vi "meas.vi"() -> ()   [LabVIEW 2010]
doc: "Use this template to create an application that executes until you click the Stop button. Unlike the Single Loop Application VI that uses polling, this VI uses the Event structure."
uses:
  <vilib>/Utility/config.llb/Read Key (String).vi
  <vilib>/Utility/config.llb/Read Key (Path).vi
  <vilib>/Utility/config.llb/Read Key (I32).vi
  <vilib>/Utility/config.llb/Read Key (Boolean).vi
  <vilib>/Utility/config.llb/Write Key (Boolean).vi
  <vilib>/Utility/config.llb/Write Key (I32).vi
  <vilib>/Utility/config.llb/Write Key (String).vi
  <vilib>/Utility/config.llb/Write Key (Path).vi
  <vilib>/Utility/config.llb/NI_LVConfig.lvlib
panel:
  in  "Export":bool
  in  "Trend":bool
  out "Array 2":u32[](array[colorbox])=[16711680, 16774656, 2783999, 65280]
  in  "MeasData":T1
  in  "Array":string[](array[string])
  in  "Tab Control":enum32{"Measurements", "View"}(tab)
  in  "Table":string[][](table)
  out "Q(R)":cluster{"Ph":i32[], dbl[]}[](graph)
  out "APD":cluster{"Ph":i32[], dbl[]}[](graph)
  out "Bar graph":cluster{"y_hist":i32[], "x_hist":i32[]}[](graph)
  out "Trend":cluster{i32[], i32[]}[](graph)
  out "Q(R)":cluster{"Ph":i32[], dbl[]}[](graph)
  out "Amplitude/Phaze":cluster{"Ph":i32[], dbl[]}[](graph)
  out "Histogram":cluster{"y_hist":i32[], "x_hist":i32[]}[](graph)
  out "ct":i32
  in  "Time delay":i32
  in  "NewFile":bool
  in  "Mesage":string(combo)
  out "Number of samples":i32
  out "ConTest":bool
  in  "VISA resource name":refnum<visa-resource-name>="ASRL1::INSTR"
  out "Connection test time":string caption="Connection test"
  in  "Stop":bool
  in  "OpenFile":bool
  in  "New":bool
  out "Object name":string
  out "File Path":path
  out "Slide":dbl(slide) scale=0.0..100.0
  in  "Auto":bool
  out "QR50":dbl[](array[numeric])
  # "Measuring"
  # "Qr50, pC"
  # "Ch 1"
  # "Ch 2"
  # "Ch 3"
  # "Ch 4"
  # "Auto"
  # "F i l e"
  # "Port name"
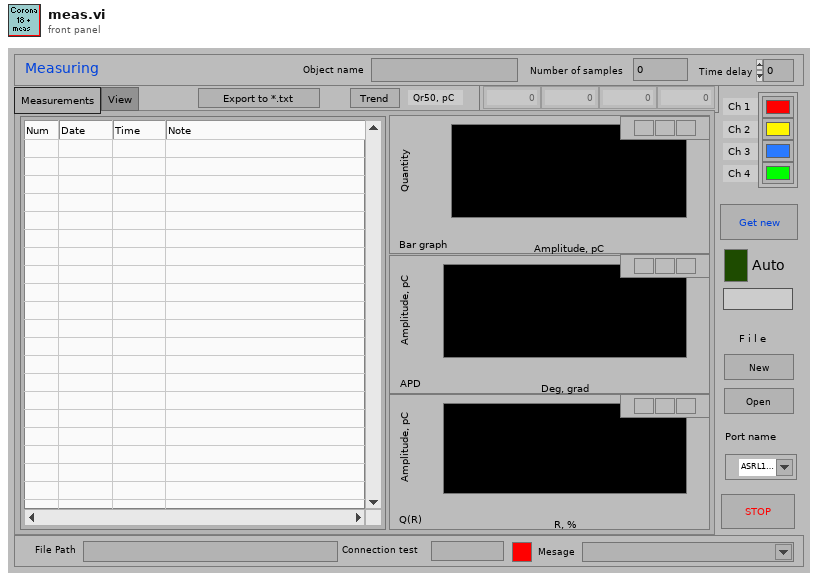
[diagram p1: front panel]
types:
  T1 = cluster{"Charge":i32, "U_Charge":i32[], "Shift":i32, "WinW":i32, "Qr":i32[][], "Ph":i32[][], "y_hist":i32[][], "x_hist":i32[][]}
  T2 = typedef "NI_LVConfig.lvlib/Config Data RefNum.ctl" = refnum<k1>
  T3 = cluster{"Array":string[], "MeasData":cluster{"Charge":i32, "U_Charge":i32[], "Shift":i32, "WinW":i32, "Qr":i32[][], "Ph":i32[][], "y_hist":i32[][], "x_hist":i32[][]}}[]
  T4 = typedef "LVRowAndColumnTypeDef.ctl" = cluster{"Row":i32, "Column":i32}
  T5 = cluster{"Array":string[], "MeasData":cluster{"Charge":i32, "U_Charge":i32[], "Shift":i32, "WinW":i32, "Qr":i32[][], "Ph":i32[][], "y_hist":i32[][], "x_hist":i32[][]}}
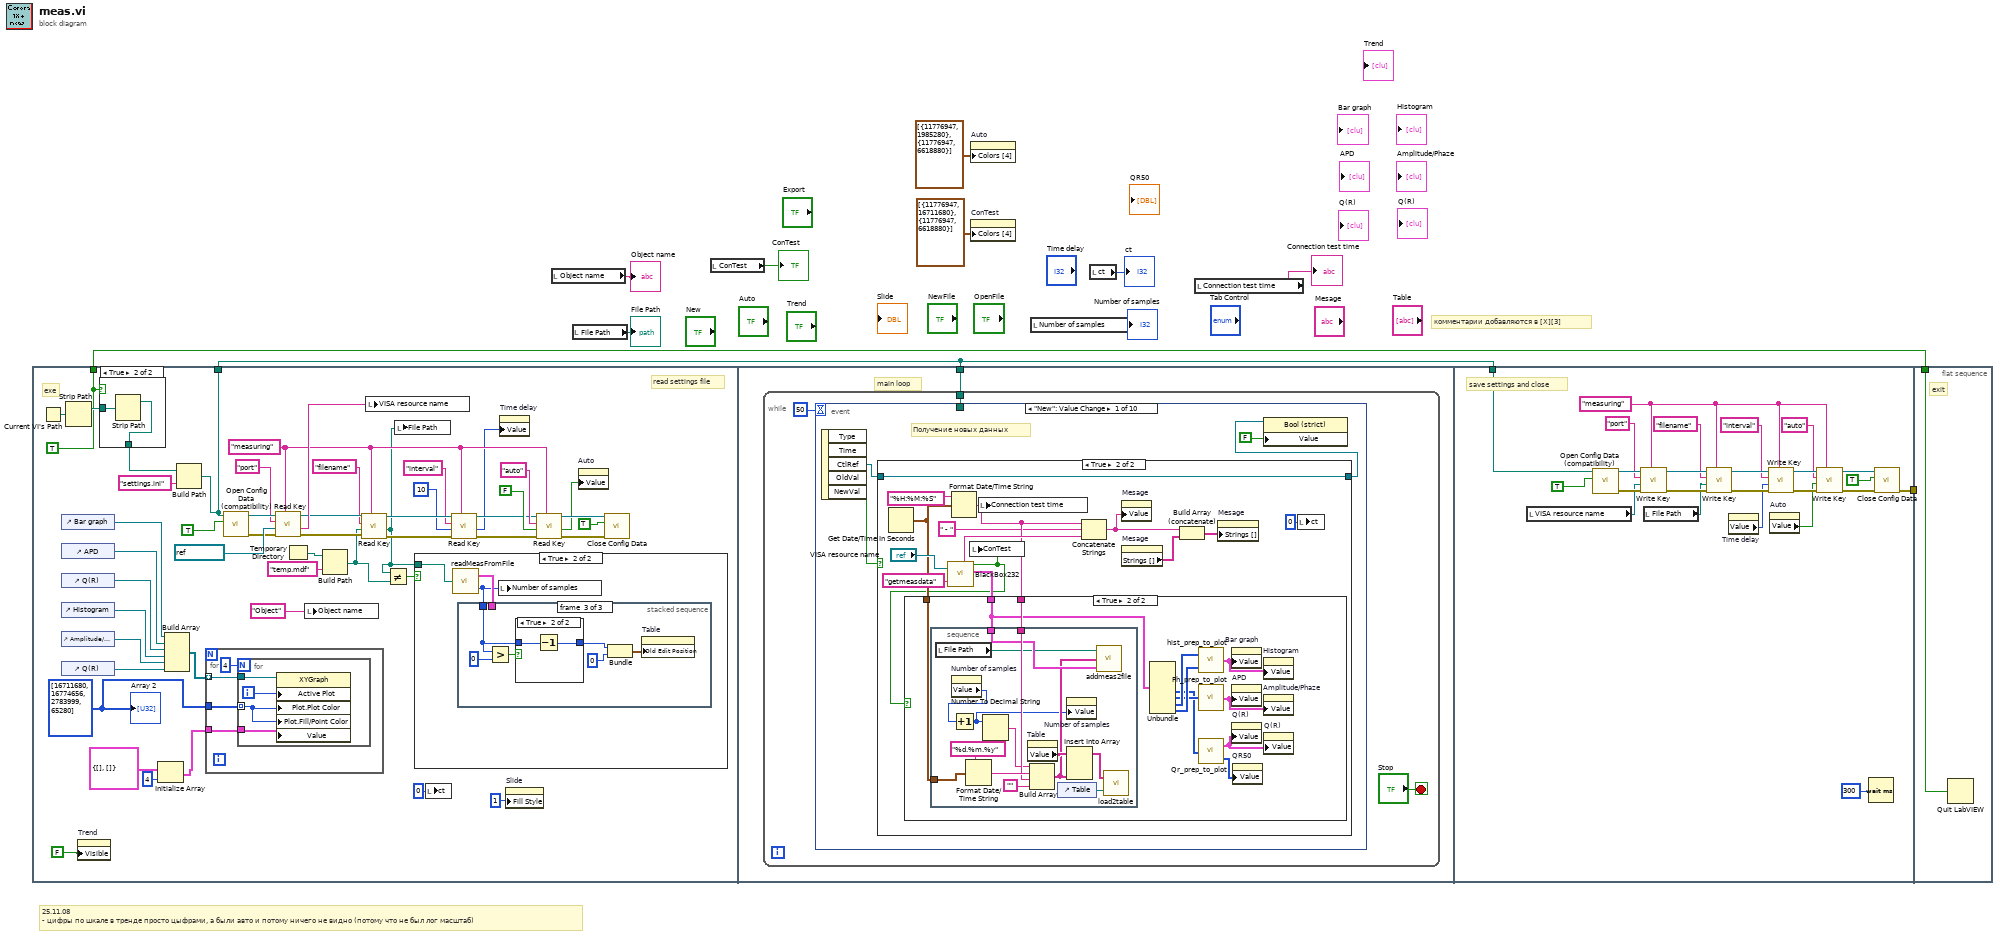
[diagram p0: block diagram]
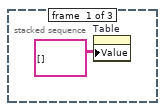
[diagram p4: hidden frame]
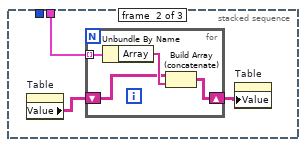
[diagram p5: hidden frame]
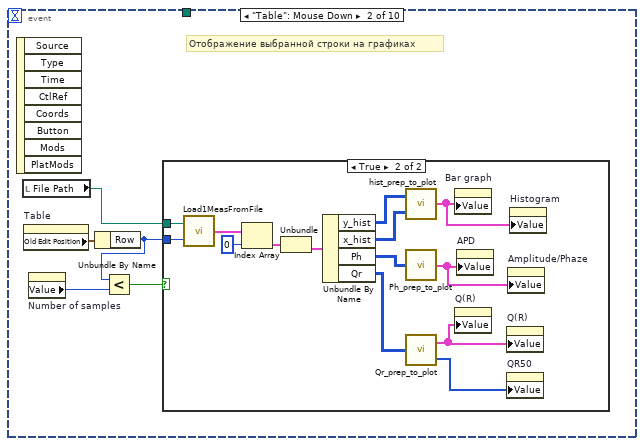
[diagram p9: hidden frame]
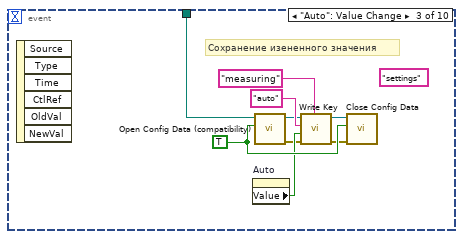
[diagram p11: hidden frame]
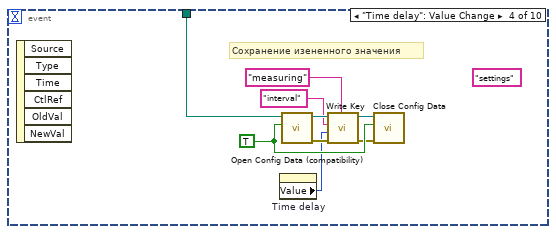
[diagram p12: hidden frame]
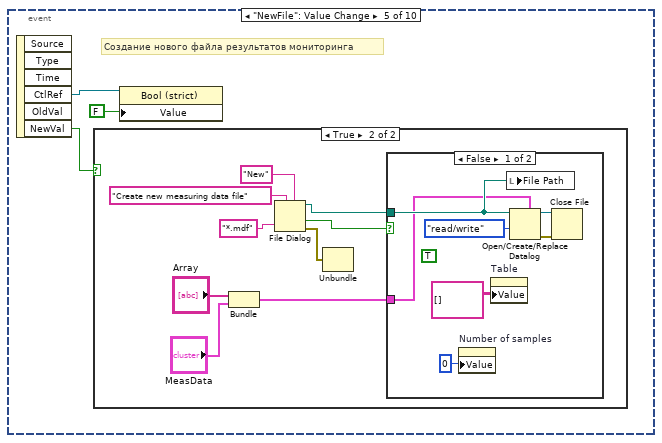
[diagram p13: hidden frame]
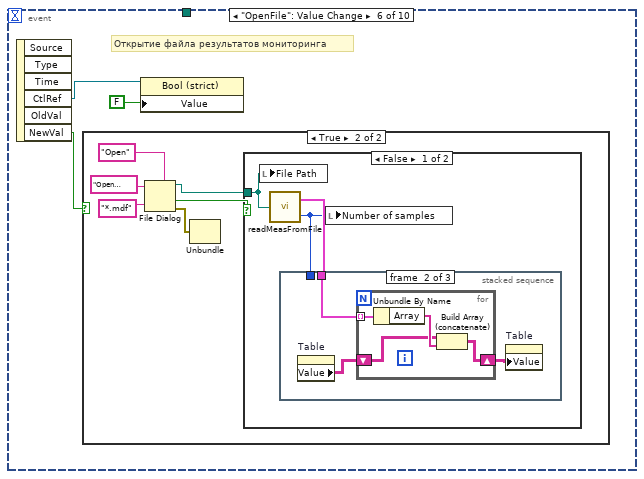
[diagram p16: hidden frame]
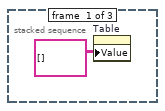
[diagram p18: hidden frame]
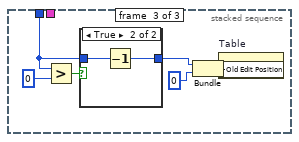
[diagram p19: hidden frame]
diagram:
  # "25.11.08\n- цифры по шкале в тренде просто цыфрами, а были авто и потому ничего не видно (потому что не был лог масштаб)"
  # "комментарии добавляются в [Х][3]"
  n1 = flat-sequence {
    tunnel: [w37] -> w3
    tunnel: [w13] -> w1
    tunnel: w3 -> [w92]
    tunnel: w3 -> [w320]
    tunnel: [w317] -> w2
    tunnel: w2 -> [_]
    tunnel: w1 -> [w341]
    frame #0 {
      w13 = TRUE ("Case Constant\n(See Context Help)")
      w20 = u32[] [16711680, 16774656, 2783999, 65280]
      w40 = "measuring" ("section")
      # "exe"
      # "read settings file"
      n2 = Current VI's Path() -> (path=w16:path)
      n3 = control-ref of="Bar graph"() -> (w25:refnum<vi>)
      n4 = control-ref of="APD"() -> (w26:refnum<vi>)
      n5 = control-ref of="Q(R)"() -> (w27:refnum<vi>)
      n6 = control-ref of="Histogram"() -> (w23:refnum<vi>)
      n7 = control-ref of="Amplitude/Phaze"() -> (w22:refnum<vi>)
      n8 = control-ref of="Q(R)"() -> (w21:refnum<vi>)
      n9 = Strip Path(path=w16) -> (stripped path=w15:path)  [unwired: 1 out]
      n10 = property on="Trend" class="XYGraph (strict)"("Visible"=FALSE) -> ()  [unwired: 2 in, 2 out]
      n11 = case shown="True" w13 {
        tunnel: w15 -> [w61 w63]
        tunnel: [w61 w62] -> w14
        frame False {
        }
        frame True {
          n12 = Strip Path(path=w63) -> (stripped path=w62:path)  [unwired: 1 out]
        }
      }
      n13 = Initialize Array(cluster{i32[], i32[]} {[], []}, 4 ("dimension size")) -> (w19:cluster{i32[], i32[]}[])
      n14 = Build Array(w25, w26, w27, w23, w22, w21) -> (w24:refnum<vi>[])
      n15 = Build Path(base path=w14, name or relative path="settings.ini") -> (appended path=w37:path)
      n16 = for {
        tunnel: w20 -> [w66]
        tunnel: w24 -> [w65] mode=indexing
        tunnel: w19 -> [w64]
        n17 = for {
          N: 4 -> [_]
          tunnel: w66 -> [w70] mode=indexing
          tunnel: w65 -> [w69]
          tunnel: w64 -> [w68]
          i -> [w71]
          n18 = property class="XYGraph"(reference=w69, "Active Plot"=w71, "Plot.Plot Color"=w70, "Plot.Fill/Point Color"=w70, "Value"=w68) -> ()  [unwired: 1 in, 2 out]
        }
      }
      n19 = call <vilib>:"Open Config Data (compatibility).vi"("create file if necessary (T)"=TRUE ("create file if necessary? (T)"), "configuration file path"=w37) -> ("error out"=w55:errorcluster, "refnum"=w58:T2)  [unwired: 7 in, 1 out]
      n20 = call-poly <vilib>:"Read Key.vi"("section"=w40, "error in (no error)"=w55, "default value"=refnum<visa-resource-name> "COM1" ("VISA resource name"), "key"="port", "refnum"=w58) -> ("error out"=w53:errorcluster, "value"=w54:string, "refnum out"=w51:T2)  [unwired: 3 in, 1 out]
      n21 = Temporary Directory() -> (w34:path)
      n22 = local write "Object name"("Object" ("Object name")) -> ()
      n23 = Build Path(base path=w34, name or relative path="temp.mdf") -> (appended path=w31:path)
      n24 = call-poly <vilib>:"Read Key.vi"("section"=w40, "error in (no error)"=w53, "default value"=w31, "key"="filename", "refnum"=w51) -> ("error out"=w52:errorcluster, "value"=w32:path, "refnum out"=w50:T2)  [unwired: 3 in, 1 out]
      n25 = local write "VISA resource name"(w54) -> ()
      n26 = Not Equal?(x=w32, y=w31) -> (x != y?=w33:bool)
      n27 = local write "File Path"(w32) -> ()
      n28 = case shown="True" w33 {
        tunnel: w32 -> [_ w72]
        frame False {
        }
        frame True {
          n29 = call "readMeasFromFile.vi"("path"=w72) -> ("data"=w74:T3, "Count"=w73:i32)
          n30 = stacked-sequence {
            tunnel: w74 -> [_ w76 _]
            tunnel: w73 -> [_ _ w84]
            frame #0 {
              n31 = property on="Table" class="Tbl (strict)"("Value"=string[][] [] ("Table")) -> ()  [unwired: 2 in, 2 out]
            }
            frame #1 {
              n32 = property on="Table" class="Tbl (strict)"() -> ("Value"=w78:string[][])  [unwired: 2 in, 2 out]
              n33 = for {
                tunnel: w76 -> [w82] mode=indexing
                shift-right: [w80] -> w77
                shift-left: w78 -> [w79]
                n34 = Unbundle By Name(w82) -> ("Array"=w81:string[])
                n35 = Build Array (concatenate)(w79, w81) -> (w80:string[][])
              }
              n36 = property on="Table" class="Tbl (strict)"("Value"=w77) -> ()  [unwired: 2 in, 2 out]
            }
            frame #2 {
              n37 = Greater?(x=w84, y=0) -> (0:w86:bool)
              n38 = case shown="True" w86 {
                tunnel: w84 -> [w89 w91]
                tunnel: [w89 w90] -> w83
                frame False {
                }
                frame True {
                  n39 = Decrement(x=w91) -> (x-1=w90:i32)
                }
              }
              n40 = Bundle("Count"=w83, 0) -> (w88:cluster{"Count":i32, i32})  [unwired: 1 in]
              n41 = property on="Table" class="Tbl (strict)"("Old Edit Position"=w88) -> ()  [unwired: 2 in, 2 out]
            }
          }
          n42 = local write "Number of samples"(w73) -> ()
        }
      }
      n43 = local write "ct"(0 ("ct")) -> ()
      n44 = call-poly <vilib>:"Read Key.vi"("section"=w40, "error in (no error)"=w52, "default value"=10, "key"="interval", "refnum"=w50) -> ("error out"=w41:errorcluster, "value"=w28:i32, "refnum out"=w44:T2)  [unwired: 3 in, 1 out]
      n45 = property on="Time delay" class="DigNum (strict)"("Value"=w28) -> ()  [unwired: 2 in, 2 out]
      n46 = property on="Slide" class="Slide (strict)"("Fill Style"=1) -> ()  [unwired: 2 in, 2 out]
      n47 = call-poly <vilib>:"Read Key.vi"("section"=w40, "error in (no error)"=w41, "default value"=FALSE, "key"="auto", "refnum"=w44) -> ("error out"=w42:errorcluster, "value"=w39:bool, "refnum out"=w43:T2)  [unwired: 3 in, 1 out]
      n48 = property on="Auto" class="Bool (strict)"("Value"=w39) -> ()  [unwired: 2 in, 2 out]
      n49 = call <vilib>:"Close Config Data.vi"("error in (no error)"=w42, "write file if changed (T)"=TRUE ("write configuration file? (T)"), "refnum"=w43) -> ()  [unwired: 7 in, 2 out]
      "Array 2" <- w20
    }
    frame #1 {
      # "main loop"
      n50 = while {
        tunnel: w92 -> [w93]
        stop <- "Stop" stop-if-true
        n51 = event shown="[0] \"New\": Value Change" {
          selector: _ -> [_ _ _ _ _ _ _ _ _ _]
          dyn-events: _ -> [_ _ _ _ _ _ _ _ _ _]
          timeout: 50 -> [_ _ _ _ _ _ _ _ _ _]
          tunnel: w93 -> [_ _ w159 w168 _ _ _ _ _ _]
          event "New": Value Change {
            # "Получение новых данных"
            n52 = event-data() -> ("CtlRef"=w97:refnum<vi>, "NewVal"=w99:bool)  [unwired: 1 in, 3 out]
            n53 = case shown="True" w99 {
              tunnel: w97 -> [w100 w102]
              tunnel: [w100 w102] -> w96
              frame False {
              }
              frame True {
                n54 = Get Date/Time In Seconds() -> (seconds since 1Jan1904=w106:timestamp)
                n55 = call "BlackBox232.vi"("Input Command"="getmeasdata", "VISA resource name"="VISA resource name") -> ("MeasData"=w103:T1, "Boolean"=w101:bool, "String"=w107:string)  [unwired: 2 out]
                n56 = Format Date/Time String(time format string (%c)="%H:%M:%S", seconds (now)=w106) -> (date/time string=w105:string)  [unwired: 1 in]
                n57 = case shown="True" w101 {
                  tunnel: w106 -> [_ w123]
                  tunnel: w105 -> [_ w122]
                  tunnel: w103 -> [_ w121]
                  frame False {
                  }
                  frame True {
                    n58 = stacked-sequence {
                      tunnel: w123 -> [w138]
                      tunnel: w122 -> [w136]
                      tunnel: w121 -> [w131]
                      frame #0 {
                        n59 = local read "File Path"() -> (w129:path)
                        n60 = property on="Number of samples" class="DigNum (strict)"() -> ("Value"=w127:i32)  [unwired: 2 in, 2 out]
                        n61 = Increment(x=w127) -> (x+1=w126:i32)
                        n62 = Format Date/Time String(time format string (%c)="%d.%m.%y", seconds (now)=w138) -> (date/time string=w137:string)  [unwired: 1 in]
                        n63 = Number To Decimal String(number=w126) -> (decimal integer string=w132:string)  [unwired: 1 in]
                        n64 = property on="Table" class="Tbl (strict)"() -> ("Value"=w135:string[][])  [unwired: 2 in, 2 out]
                        n65 = Build Array(w132, w137, w136, "" ("element")) -> (w130:string[])
                        n66 = control-ref of="Table"() -> (w133:refnum<vi>)
                        n67 = property on="Number of samples" class="DigNum (strict)"("Value"=w126) -> ()  [unwired: 2 in, 2 out]
                        n68 = Insert Into Array(array=w135, new element=w130) -> (w134:string[][])  [unwired: 2 in]
                        n69 = call "addmeas2file.vi"("MeasData"=w131, "Array"=w130, "File Path"=w129) -> ()
                        n70 = call "load2table.vi"("Table"=w133, "Array"=w134) -> ()  [unwired: 1 out]
                      }
                    }
                    n71 = Unbundle(w121) -> ("Qr"=w119:i32[][], "Ph"=w120:i32[][], "y_hist"=w125:i32[][], "x_hist"=w124:i32[][])  [unwired: 4 out]
                    n72 = call "hist_prep_to_plot.vi"("x_hist"=w124, "y_hist"=w125) -> ("Array"=w118:cluster{"y_hist":i32[], "x_hist":i32[]}[])
                    n73 = call "Ph_prep_to_plot.vi"("Ph"=w120) -> ("Array"=w117:cluster{"Ph":i32[], dbl[]}[])
                    n74 = call "Qr_prep_to_plot.vi"("Qr"=w119) -> ("Array"=w116:cluster{"Ph":i32[], dbl[]}[], "QR50"=w115:i32[])
                    n75 = property on="Bar graph" class="XYGraph (strict)"("Value"=w118) -> ()  [unwired: 2 in, 2 out]
                    n76 = property on="APD" class="XYGraph (strict)"("Value"=w117) -> ()  [unwired: 2 in, 2 out]
                    n77 = property on="Q(R)" class="XYGraph (strict)"("Value"=w116) -> ()  [unwired: 2 in, 2 out]
                    n78 = property on="QR50" class="Arr (strict)"("Value"=w115) -> ()  [unwired: 2 in, 2 out]
                    n79 = property on="Histogram" class="XYGraph (strict)"("Value"=w118) -> ()  [unwired: 2 in, 2 out]
                    n80 = property on="Amplitude/Phaze" class="XYGraph (strict)"("Value"=w117) -> ()  [unwired: 2 in, 2 out]
                    n81 = property on="Q(R)" class="XYGraph (strict)"("Value"=w116) -> ()  [unwired: 2 in, 2 out]
                  }
                }
                n82 = local write "ConTest"(w101) -> ()
                n83 = local write "Connection test time"(w105) -> ()
                n84 = Concatenate Strings(w105, " - ", w107) -> (w108:string)
                n85 = property on="Mesage" class="CmbBox"("Value"=w108) -> ()  [unwired: 2 in, 2 out]
                n86 = property on="Mesage" class="CmbBox"() -> ("Strings []"=w110:string[])  [unwired: 2 in, 2 out]
                n87 = Build Array (concatenate)(w108, w110) -> (w109:string[])
                n88 = property on="Mesage" class="CmbBox"("Strings []"=w109) -> ()  [unwired: 2 in, 2 out]
                n89 = local write "ct"(0 ("ct")) -> ()
              }
            }
            n90 = property class="Bool (strict)"(reference=w96, "Value"=FALSE) -> ()  [unwired: 1 in, 2 out]
          }
          event "Table": Mouse Down {
            # "Отображение выбранной строки на графиках"
            n91 = event-data() -> ()  [unwired: 1 in, 8 out]
            n92 = local read "File Path"() -> (w143:path)
            n93 = property on="Table" class="Tbl (strict)"() -> ("Old Edit Position"=w144:T4)  [unwired: 2 in, 2 out]
            n94 = property on="Number of samples" class="DigNum (strict)"() -> ("Value"=w140:i32)  [unwired: 2 in, 2 out]
            n95 = Unbundle By Name(w144) -> ("Row"=w141:i32)
            n96 = Less?(x=w141, y=w140) -> (x < y?=w142:bool)
            n97 = case shown="True" w142 {
              tunnel: w143 -> [_ w158]
              tunnel: w141 -> [_ w157]
              frame False {
              }
              frame True {
                n98 = call "Load1MeasFromFile.vi"("Index"=w157, "path"=w158) -> ("data"=w156:T3)
                n99 = Index Array(array=w156, index=0) -> (element=w154:T5)
                n100 = Unbundle(w154) -> ("MeasData"=w153:T1)  [unwired: 1 out]
                n101 = Unbundle By Name(w153) -> ("y_hist"=w152:i32[][], "x_hist"=w151:i32[][], "Ph"=w150:i32[][], "Qr"=w146:i32[][])
                n102 = call "hist_prep_to_plot.vi"("x_hist"=w151, "y_hist"=w152) -> ("Array"=w147:cluster{"y_hist":i32[], "x_hist":i32[]}[])
                n103 = call "Ph_prep_to_plot.vi"("Ph"=w150) -> ("Array"=w148:cluster{"Ph":i32[], dbl[]}[])
                n104 = call "Qr_prep_to_plot.vi"("Qr"=w146) -> ("Array"=w149:cluster{"Ph":i32[], dbl[]}[], "QR50"=w145:i32[])
                n105 = property on="Bar graph" class="XYGraph (strict)"("Value"=w147) -> ()  [unwired: 2 in, 2 out]
                n106 = property on="Q(R)" class="XYGraph (strict)"("Value"=w149) -> ()  [unwired: 2 in, 2 out]
                n107 = property on="APD" class="XYGraph (strict)"("Value"=w148) -> ()  [unwired: 2 in, 2 out]
                n108 = property on="Q(R)" class="XYGraph (strict)"("Value"=w149) -> ()  [unwired: 2 in, 2 out]
                n109 = property on="QR50" class="Arr (strict)"("Value"=w145) -> ()  [unwired: 2 in, 2 out]
                n110 = property on="Amplitude/Phaze" class="XYGraph (strict)"("Value"=w148) -> ()  [unwired: 2 in, 2 out]
                n111 = property on="Histogram" class="XYGraph (strict)"("Value"=w147) -> ()  [unwired: 2 in, 2 out]
              }
            }
          }
          event "Auto": Value Change {
            (unwired) "settings" ("section")
            w167 = TRUE ("create file if necessary? (T)")
            # "Сохранение изененного значения"
            n112 = event-data() -> ()  [unwired: 1 in, 6 out]
            n113 = property on="Auto" class="Bool (strict)"() -> ("Value"=w166:bool)  [unwired: 2 in, 2 out]
            n114 = call <vilib>:"Open Config Data (compatibility).vi"("create file if necessary (T)"=w167, "configuration file path"=w159) -> ("error out"=w164:errorcluster, "refnum"=w160:T2)  [unwired: 7 in, 1 out]
            n115 = call-poly <vilib>:"Write Key.vi"("section"="measuring", "error in (no error)"=w164, "value"=w166, "key"="auto", "refnum"=w160) -> ("error out"=w165:errorcluster, "refnum out"=w161:T2)  [unwired: 4 in, 1 out]
            n116 = call <vilib>:"Close Config Data.vi"("error in (no error)"=w165, "write file if changed (T)"=w167, "refnum"=w161) -> ()  [unwired: 7 in, 2 out]
          }
          event "Time delay": Value Change {
            (unwired) "settings" ("section")
            w176 = TRUE ("create file if necessary? (T)")
            # "Сохранение изененного значения"
            n117 = event-data() -> ()  [unwired: 1 in, 6 out]
            n118 = property on="Time delay" class="DigNum (strict)"() -> ("Value"=w169:i32)  [unwired: 2 in, 2 out]
            n119 = call <vilib>:"Open Config Data (compatibility).vi"("create file if necessary (T)"=w176, "configuration file path"=w168) -> ("error out"=w174:errorcluster, "refnum"=w171:T2)  [unwired: 7 in, 1 out]
            n120 = call-poly <vilib>:"Write Key.vi"("section"="measuring", "error in (no error)"=w174, "value"=w169, "key"="interval", "refnum"=w171) -> ("error out"=w175:errorcluster, "refnum out"=w172:T2)  [unwired: 4 in, 1 out]
            n121 = call <vilib>:"Close Config Data.vi"("error in (no error)"=w175, "write file if changed (T)"=w176, "refnum"=w172) -> ()  [unwired: 7 in, 2 out]
          }
          event "NewFile": Value Change {
            # "Создание нового файла результатов мониторинга"
            n122 = event-data() -> ("CtlRef"=w178:refnum<vi>, "NewVal"=w179:bool)  [unwired: 1 in, 4 out]
            n123 = case shown="True" w179 {
              frame False {
              }
              frame True {
                n124 = Bundle("Array"="Array", "MeasData"="MeasData") -> (w181:T5)  [unwired: 1 in]
                n125 = File Dialog(5:"New" ("button label"), 6:"*.mdf" ("pattern"), 7:"Create new measuring data file" ("prompt")) -> (0:w180:errorcluster, 1:w187:bool, 3:w186:path)  [unwired: 4 in, 1 out]
                n126 = Unbundle(w180) -> ()  [unwired: 3 out]
                n127 = case shown="False" w187 {
                  tunnel: w186 -> [w195 _]
                  tunnel: w181 -> [w192 _]
                  frame False {
                    (unwired) TRUE ("overwrite (F)")
                    n128 = property on="Number of samples" class="DigNum (strict)"("Value"=0 ("Number of samples")) -> ()  [unwired: 2 in, 2 out]
                    n129 = property on="Table" class="Tbl (strict)"("Value"=string[][] [] ("Table")) -> ()  [unwired: 2 in, 2 out]
                    n130 = local write "File Path"(w195) -> ()
                    n131 = Open/Create/Replace Datalog(5:w192, 9:enum16{"read/write", "read-only", "write-only"}."read/write" ("access (0:read/write)"), 11:w195) -> (0:w194:errorcluster, 3:w193:refnum<k1>)  [unwired: 3 in, 1 out]
                    n132 = Close File(refnum=w193, error in=w194) -> ()  [unwired: 2 out]
                  }
                  frame True {
                  }
                }
              }
            }
            n133 = property class="Bool (strict)"(reference=w178, "Value"=FALSE) -> ()  [unwired: 1 in, 2 out]
          }
          event "OpenFile": Value Change {
            # "Открытие файла результатов мониторинга"
            n134 = event-data() -> ("CtlRef"=w197:refnum<vi>, "NewVal"=w198:bool)  [unwired: 1 in, 4 out]
            n135 = case shown="True" w198 {
              frame False {
              }
              frame True {
                n136 = File Dialog(5:"Open" ("button label"), 6:"*.mdf" ("pattern"), 7:"Open measuring data file " ("prompt")) -> (0:w199:errorcluster, 1:w201:bool, 3:w200:path)  [unwired: 4 in, 1 out]
                n137 = Unbundle(w199) -> ()  [unwired: 3 out]
                n138 = case shown="False" w201 {
                  tunnel: w200 -> [w207 _]
                  frame False {
                    n139 = local write "File Path"(w207) -> ()
                    n140 = call "readMeasFromFile.vi"("path"=w207) -> ("data"=w206:T3, "Count"=w205:i32)
                    n141 = stacked-sequence {
                      tunnel: w206 -> [_ w209 _]
                      tunnel: w205 -> [_ _ w217]
                      frame #0 {
                        n142 = property on="Table" class="Tbl (strict)"("Value"=string[][] [] ("Table")) -> ()  [unwired: 2 in, 2 out]
                      }
                      frame #1 {
                        n143 = property on="Table" class="Tbl (strict)"() -> ("Value"=w211:string[][])  [unwired: 2 in, 2 out]
                        n144 = for {
                          tunnel: w209 -> [w215] mode=indexing
                          shift-right: [w213] -> w210
                          shift-left: w211 -> [w212]
                          n145 = Unbundle By Name(w215) -> ("Array"=w214:string[])
                          n146 = Build Array (concatenate)(w212, w214) -> (w213:string[][])
                        }
                        n147 = property on="Table" class="Tbl (strict)"("Value"=w210) -> ()  [unwired: 2 in, 2 out]
                      }
                      frame #2 {
                        n148 = Greater?(x=w217, y=0) -> (0:w219:bool)
                        n149 = case shown="True" w219 {
                          tunnel: w217 -> [w222 w224]
                          tunnel: [w222 w223] -> w216
                          frame False {
                          }
                          frame True {
                            n150 = Decrement(x=w224) -> (x-1=w223:i32)
                          }
                        }
                        n151 = Bundle("Count"=w216, 0) -> (w221:cluster{"Count":i32, i32})  [unwired: 1 in]
                        n152 = property on="Table" class="Tbl (strict)"("Old Edit Position"=w221) -> ()  [unwired: 2 in, 2 out]
                      }
                    }
                    n153 = local write "Number of samples"(w205) -> ()
                  }
                  frame True {
                  }
                }
              }
            }
            n154 = property class="Bool (strict)"(reference=w197, "Value"=FALSE) -> ()  [unwired: 1 in, 2 out]
          }
          event Timeout {
            w225 = FALSE ("Case Constant\n(See Context Help) 2")
            # "Таймаут - просто мигалка если true  и шедулер если false"
            n155 = event-data() -> ()  [unwired: 1 in, 3 out]
            n156 = Not(x=w225) -> (.not. x?=w226:bool)
            n157 = case shown="False" w225 {
              frame False {
              }
              frame True {
                n158 = control-ref of="Slide"() -> (w249:refnum<vi>)
                n159 = property class="Slide (strict)"(reference=w249) -> (reference out=w244:refnum<vi>, "Value"=w245:dbl, "Fill Style"=w243:i32)  [unwired: 1 in, 1 out]
                n160 = Greater?(x=w245, y=100.0) -> (0:w247:bool)
                n161 = case shown="True" w247 {
                  tunnel: [w252 0.0] -> w246
                  tunnel: w245 -> [w251 _]
                  tunnel: w243 -> [w250 w254]
                  tunnel: [w250 w253] -> w242
                  frame False {
                    n162 = Increment(x=w251) -> (x+1=w252:dbl)
                  }
                  frame True {
                    n163 = case shown="1, Default" w254 {
                      tunnel: [2 1] -> w253
                      frame 1, Default {
                      }
                      frame 2 {
                      }
                    }
                  }
                }
                n164 = property class="Slide (strict)"(reference=w244, "Value"=w246, "Fill Style"=w242) -> ()  [unwired: 1 in, 2 out]
              }
            }
            n165 = case shown="True" w226 {
              frame False {
              }
              frame True {
                n166 = property on="Time delay" class="DigNum (strict)"() -> ("Value"=w227:i32)  [unwired: 2 in, 2 out]
                n167 = expression code="x*1200"(w227) -> (w231:i32)
                n168 = local read "ct"() -> (w228:i32)
                n169 = Greater?(x=w228, y=w231) -> (0:w230:bool)
                n170 = case shown="True" w230 {
                  tunnel: [w232 0] -> w229
                  tunnel: w228 -> [w234 _]
                  tunnel: w227 -> [w233 _]
                  frame False {
                    n171 = Increment(x=w234) -> (x+1=w236:i32)
                    n172 = local write "ct"(w236) -> ()
                    n173 = expression code="x/12"(w236) -> (w235:i32)
                    n174 = Divide(x=w235, y=w233) -> (x/y=w232:dbl)
                  }
                  frame True {
                    n175 = property on="Auto" class="Bool (strict)"() -> ("Value"=w237:bool)  [unwired: 2 in, 2 out]
                    n176 = local write "ct"(0 ("ct")) -> ()
                    n177 = case shown="True" w237 {
                      frame False {
                      }
                      frame True {
                        n178 = control-ref of="New"() -> (w240:refnum<vi>)
                        n179 = property class="Bool (strict)"(reference=w240, "Value (Signaling)"=TRUE ("New")) -> ()  [unwired: 1 in, 2 out]
                      }
                    }
                  }
                }
                n180 = property on="Slide" class="Slide (strict)"("Value"=w229) -> ()  [unwired: 2 in, 2 out]
              }
            }
          }
          event "Table": Value Change {
            # "Изменение значений в таблице\nНовые значения из столбика \"комментарии\" будут сохранены в файл"
            n181 = event-data() -> ("NewVal"=w263:string[][])  [unwired: 1 in, 5 out]
            n182 = property on="Table" class="Tbl (strict)"() -> ("Old Edit Position"=w267:T4)  [unwired: 2 in, 2 out]
            n183 = local read "File Path"() -> (w264:path)
            n184 = property on="Number of samples" class="DigNum (strict)"() -> ("Value"=w266:i32)  [unwired: 2 in, 2 out]
            n185 = Unbundle By Name(w267) -> ("Row"=w265:i32, "Column"=w258:i32)
            n186 = Less?(x=w265, y=w266) -> (x < y?=w261:bool)
            n187 = Equal?(x=w258, y=3) -> (x = y?=w260:bool)
            n188 = And(x=w260, y=w261) -> (x .and. y?=w262:bool)
            n189 = case shown="True" w262 {
              tunnel: w265 -> [_ w271]
              tunnel: w264 -> [_ w278]
              tunnel: w263 -> [_ w272]
              frame False {
              }
              frame True {
                n190 = call "Load1MeasFromFile.vi"("Index"=w271, "path"=w278) -> ("data"=w281:T3)
                n191 = Index Array(array=w281, index=0) -> (element=w279:T5)
                n192 = Unbundle(w279) -> ("Array"=w276:string[], "MeasData"=w277:T1)
                n193 = Index Array(array=w272, index (row)=w271, index (col)=3 ("disabled index (col)")) -> (element=w269:string)
                n194 = Decimate 1D Array(w276) -> (w275:string[], w274:string[], w273:string[])  [unwired: 1 out]
                n195 = Build Array (concatenate)(w275, w274, w273, w269) -> (w268:string[])
                n196 = call "insmeas2file.vi"("Numeric"=w271, "MeasData"=w277, "Array"=w268, "File Path"=w278) -> ()  [unwired: 1 out]
              }
            }
          }
          event "Trend": Value Change {
            n197 = event-data() -> ("NewVal"=w282:bool)  [unwired: 1 in, 5 out]
            n198 = property on="Trend" class="XYGraph (strict)"("Visible"=w282) -> ()  [unwired: 2 in, 2 out]
            n199 = case shown="True" w282 {
              frame False {
              }
              frame True {
                w293 = i32[] []
                n200 = local read "File Path"() -> (w295:path)
                n201 = call "readMeasFromFile.vi"("path"=w295) -> ("data"=w294:T3)  [unwired: 1 out]
                n202 = for {
                  tunnel: w294 -> [w314] mode=indexing
                  shift-right: [w309] -> w288
                  shift-left: w293 -> [w310]
                  shift-right: [w307] -> w289
                  shift-left: w293 -> [w306]
                  shift-right: [w308] -> w290
                  shift-left: w293 -> [w303]
                  shift-right: [w300] -> w291
                  shift-left: w293 -> [w301]
                  shift-right: [w299] -> w292
                  shift-left: w293 -> [w298]
                  i -> [w297]
                  n203 = Unbundle By Name(w314) -> ("MeasData.Qr"=w313:i32[][])
                  n204 = call "Qr_prep_to_plot.vi"("Qr"=w313) -> ("QR50"=w312:i32[])  [unwired: 1 out]
                  n205 = call "14to41.vi"("QR50"=w312) -> ("0"=w311:i32, "1"=w305:i32, "2"=w304:i32, "3"=w302:i32)
                  n206 = Increment(x=w297) -> (x+1=w296:i32)
                  n207 = Build Array (concatenate)(w306, w305) -> (w307:i32[])
                  n208 = Build Array (concatenate)(w303, w304) -> (w308:i32[])
                  n209 = Build Array (concatenate)(w301, w302) -> (w300:i32[])
                  n210 = Build Array (concatenate)(w310, w311) -> (w309:i32[])
                  n211 = Build Array (concatenate)(w298, w296) -> (w299:i32[])
                }
                n212 = Bundle(w292, w288) -> (w284:cluster{i32[], i32[]})  [unwired: 1 in]
                n213 = Bundle(w292, w289) -> (w287:cluster{i32[], i32[]})  [unwired: 1 in]
                n214 = Bundle(w292, w290) -> (w286:cluster{i32[], i32[]})  [unwired: 1 in]
                n215 = Bundle(w292, w291) -> (w285:cluster{i32[], i32[]})  [unwired: 1 in]
                n216 = Build Array(w284, w287, w286, w285) -> (w283:cluster{i32[], i32[]}[])
                n217 = property on="Trend" class="XYGraph (strict)"("Value"=w283) -> ()  [unwired: 2 in, 2 out]
              }
            }
          }
          event "Export": Value Change {
            # "Экспорт файла данных в текстовый формат"
            n218 = event-data() -> ("NewVal"=w315:bool)  [unwired: 1 in, 5 out]
            n219 = case shown="True" w315 {
              frame False {
              }
              frame True {
                n220 = local read "File Path"() -> (w316:path)
                n221 = call "ExportMeas2TXT1.vi"("File Path"=w316) -> ()  [unwired: 1 out]
              }
            }
          }
        }
      }
    }
    frame #2 {
      w327 = "measuring" ("section")
      # "save settings and close"
      n222 = local read "VISA resource name"() -> (w335:refnum<visa-resource-name>)
      n223 = call <vilib>:"Open Config Data (compatibility).vi"("create file if necessary (T)"=TRUE ("create file if necessary? (T)"), "configuration file path"=w320) -> ("error out"=w338:errorcluster, "refnum"=w340:T2)  [unwired: 7 in, 1 out]
      n224 = call-poly <vilib>:"Write Key.vi"("section"=w327, "error in (no error)"=w338, "value"=w335, "key"="port", "refnum"=w340) -> ("error out"=w331:errorcluster, "refnum out"=w334:T2)  [unwired: 4 in, 1 out]
      n225 = local read "File Path"() -> (w328:path)
      n226 = call-poly <vilib>:"Write Key.vi"("section"=w327, "error in (no error)"=w331, "value"=w328, "key"="filename", "refnum"=w334) -> ("error out"=w332:errorcluster, "refnum out"=w333:T2)  [unwired: 4 in, 1 out]
      n227 = property on="Time delay" class="DigNum (strict)"() -> ("Value"=w318:i32)  [unwired: 2 in, 2 out]
      n228 = call-poly <vilib>:"Write Key.vi"("section"=w327, "error in (no error)"=w332, "value"=w318, "key"="interval", "refnum"=w333) -> ("error out"=w325:errorcluster, "refnum out"=w326:T2)  [unwired: 4 in, 1 out]
      n229 = property on="Auto" class="Bool (strict)"() -> ("Value"=w321:bool)  [unwired: 2 in, 2 out]
      n230 = call-poly <vilib>:"Write Key.vi"("section"=w327, "error in (no error)"=w325, "value"=w321, "key"="auto", "refnum"=w326) -> ("error out"=w324:errorcluster, "refnum out"=w323:T2)  [unwired: 4 in, 1 out]
      n231 = Wait (ms)(milliseconds to wait=u32 300) -> ()  [unwired: 1 out]
      n232 = call <vilib>:"Close Config Data.vi"("error in (no error)"=w324, "write file if changed (T)"=TRUE ("write configuration file? (T)"), "refnum"=w323) -> ("error out"=w317:errorcluster)  [unwired: 7 in, 1 out]
    }
    frame #3 {
      # "exit"
      n233 = Quit LabVIEW(quit? (T)=w341) -> ()
    }
  }
  n234 = local read "Object name"() -> (→"Object name":string)
  n235 = local read "File Path"() -> (→"File Path":path)
  n236 = local read "ConTest"() -> (→"ConTest":bool)
  n237 = property on="Auto" class="Bool (strict)"("Colors [4]"=cluster{u32, u32}[] [{11776947, 1985280}, {11776947, 6618880}]) -> ()  [unwired: 2 in, 2 out]
  n238 = property on="ConTest" class="Bool (strict)"("Colors [4]"=cluster{u32, u32}[] [{11776947, 16711680}, {11776947, 6618880}]) -> ()  [unwired: 2 in, 2 out]
  n239 = local read "Number of samples"() -> (→"Number of samples":i32)
  n240 = local read "ct"() -> (→"ct":i32)
  n241 = local read "Connection test time"() -> (→"Connection test time":string)
